vi "no timeout error.vi"(1 "error in (no error)":errorcluster) -> (0 "error out":errorcluster)   [LabVIEW 2011]
doc: "When an error code is equal to 56 (time out error), the error cluster is initialized to 0 (no error)."
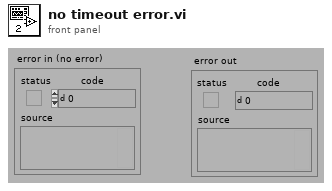
[diagram p1: front panel]
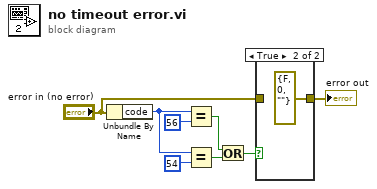
[diagram p0: block diagram]
diagram:
  n1 = Unbundle By Name("error in (no error)") -> ("code"=w2:i32)
  n2 = Equal?(x=w2, y=56) -> (x = y?=w5:bool)
  n3 = Equal?(x=w2, y=54) -> (x = y?=w4:bool)
  n4 = Or(x=w5, y=w4) -> (x .or. y?=w1:bool)
  n5 = case shown="True" w1 {
    tunnel: "error in (no error)" -> [w9 _]
    tunnel: [w9 errorcluster {"status"=FALSE, "code"=0, "source"=""} ("error out")] -> w6
    frame False {
    }
    frame True {
    }
  }
  "error out" <- w6
